vi "SL2_AD_DLL_Phoibos_GetVoltageRange.vi"(6 "error in":errorcluster, 7 "voltage_name":string, 8 "pHandle":u32, 9 "dll path in":path) -> (0 "error out":errorcluster, 1 "min":dbl, 2 "max":dbl, 3 "dll path out":path)   [LabVIEW 2020]
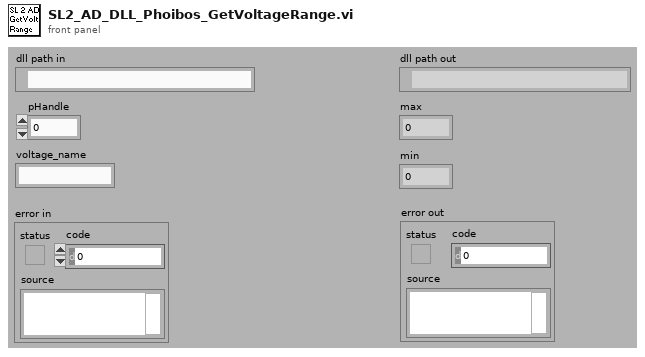
[diagram p1: front panel]
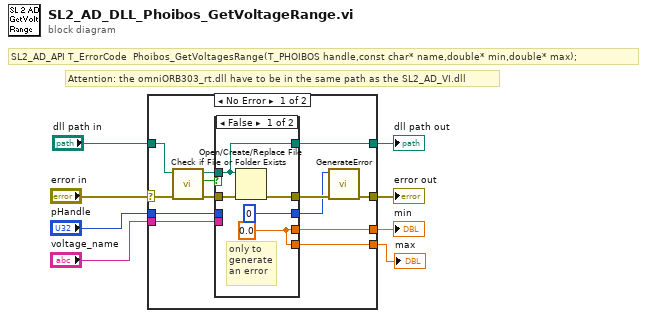
[diagram p0: block diagram]
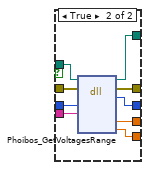
[diagram p2: hidden frame]
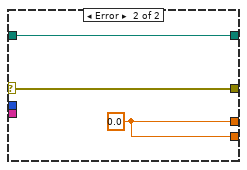
[diagram p3: hidden frame]
diagram:
  # "SL2_AD_API T_ErrorCode  Phoibos_GetVoltagesRange(T_PHOIBOS handle,const char* name,double* min,double* max);"
  # "Attention: the omniORB303_rt.dll have to be in the same path as the SL2_AD_VI.dll"
  n1 = case shown="No Error" "error in" {
    selector: "error in" -> [w20 w37]
    tunnel: [w13 w37] -> w8
    tunnel: [w21 w38] -> w7
    tunnel: "dll path in" -> [w19 w38]
    tunnel: "voltage_name" -> [w18 _]
    tunnel: "pHandle" -> [w17 _]
    tunnel: [w16 w36] -> w2
    tunnel: [w15 w36] -> w1
    frame No Error {
      n2 = call <vilib>:"Check if File or Folder Exists.vi"("error in (no error)"=w20, "path"=w19) -> ("error out"=w9:errorcluster, "file or folder exists?"=w11:bool, "dup path"=w10:path)  [unwired: 7 in]
      n3 = case shown="False" w11 {
        tunnel: [w25 w35] -> w14
        tunnel: [u32 0 ("error_code") w34] -> w12
        tunnel: [w24 w33] -> w21
        tunnel: w10 -> [w24 w32]
        tunnel: w9 -> [w26 w31]
        tunnel: w18 -> [_ w30]
        tunnel: w17 -> [_ w29]
        tunnel: [w22 w28] -> w16
        tunnel: [w22 w27] -> w15
        frame False {
          w22 = 0.0 ("min")
          # "only to generate an error"
          n4 = Open/Create/Replace File(file path (use dialog)=w24, error in=w26) -> (error out=w25:errorcluster)  [unwired: 4 in, 2 out]
        }
        frame True {
          n5 = dll-call lib="C:/Programme/SPECS/SpecsLab2/programming/LabView7.1/SL2_AD_VI.dll" fn="Phoibos_GetVoltagesRange" ("GetVoltageRange")(path in=w32, error in=w31, "handle"=w29, "voltage_name"=w30) -> (path out=w33:path, error out=w35:errorcluster, "error_code"=w34:u32, "min"=w28:dbl, "max"=w27:dbl)  [unwired: 5 in]
        }
      }
      n6 = call "GenerateError.vi"("error in"=w14, "error_code"=w12) -> ("error out"=w13:errorcluster)  [unwired: 9 in]
    }
    frame Error {
      w36 = 0.0 ("max")
    }
  }
  "error out" <- w8
  "dll path out" <- w7
  "min" <- w2
  "max" <- w1
